vi "ParseAnemoString.vi"(11 "String":string) -> (0 "error out":errorcluster, 2 "direction":dbl, 3 "speed":dbl)   [LabVIEW 2011]
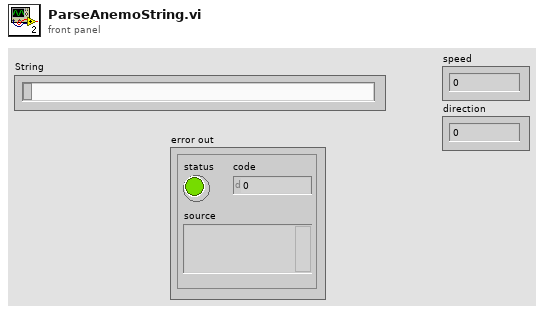
[diagram p1: front panel]
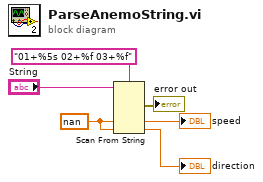
[diagram p0: block diagram]
diagram:
  w1 = nan ("default value 2")
  n1 = Scan From String(format string="01+%5s 02+%f 03+%f", input string="String", default 2=w1, default 3=w1) -> (error out=→"error out":errorcluster, output 2=→"speed":dbl, output 3=→"direction":dbl)  [unwired: 4 in, 2 out]
